vi "HipEXO_SM_R.vi"(10 "Trigger Ratio":dbl, 11 "Hip Angle":dbl) -> (1 "Flexion":bool, 2 "Extension":bool, 3 "ROM":dbl)   [LabVIEW 2018]
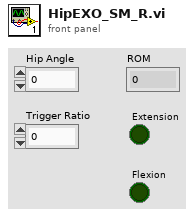
[diagram p1: front panel]
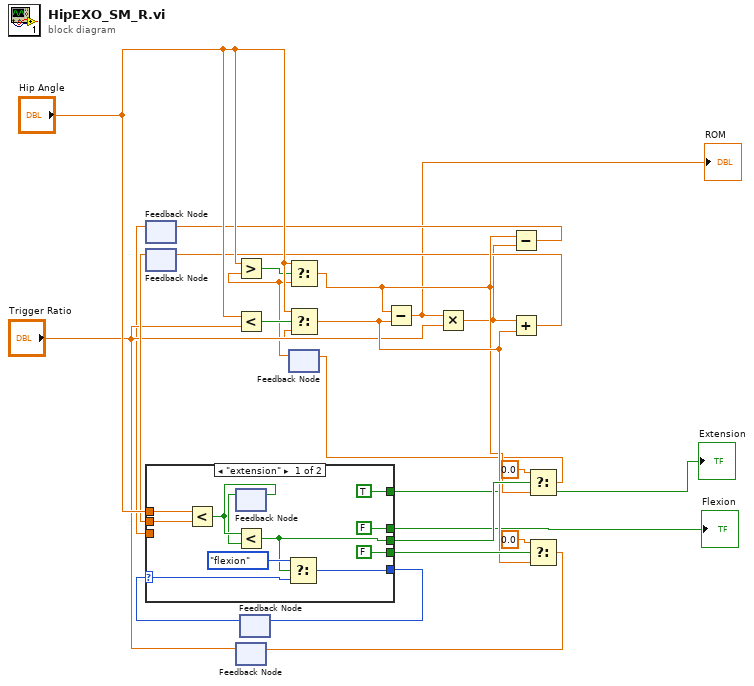
[diagram p0: block diagram]
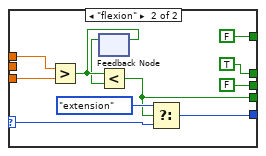
[diagram p2: hidden frame]
diagram:
  n1 = feedback #1() -> (w1:dbl)  [unwired: 1 in]
  n2 = feedback #2() -> (w16:dbl)  [unwired: 1 in]
  n3 = feedback #3() -> (w10:dbl)  [unwired: 1 in]
  n4 = Less?(x="Hip Angle", y=w10) -> (x < y?=w7:bool)
  n5 = feedback #4() -> (w3:enum16{"flexion", "extension"})  [unwired: 1 in]
  n6 = case shown="\"extension\"" w3 {
    selector: w3 -> [w32 w43]
    tunnel: [TRUE FALSE] -> w18
    tunnel: [w33 w44] -> w2
    tunnel: [FALSE TRUE] -> w19
    tunnel: "Hip Angle" -> [w30 w41]
    tunnel: w16 -> [w29 _]
    tunnel: w1 -> [_ w40]
    tunnel: [w25 FALSE ("output")] -> w22
    tunnel: [FALSE ("output") w36] -> w23
    frame "extension" {
      n7 = Less?(x=w30, y=w29) -> (x < y?=w27:bool)
      n8 = feedback-in #5(w27) -> ()
      n9 = feedback #5() -> (w26:bool)  [unwired: 1 in]
      n10 = Less?(x=w27, y=w26) -> (x < y?=w25:bool)
      n11 = Select(t=enum16{"flexion", "extension"}."flexion", s=w25, f=w32) -> (s? t:f=w33:enum16{"flexion", "extension"})
    }
    frame "flexion" {
      n12 = Greater?(x=w41, y=w40) -> (0:w38:bool)
      n13 = feedback-in #6(w38) -> ()
      n14 = feedback #6() -> (w37:bool)  [unwired: 1 in]
      n15 = Less?(x=w38, y=w37) -> (x < y?=w36:bool)
      n16 = Select(t=enum16{"flexion", "extension"}."extension", s=w36, f=w43) -> (s? t:f=w44:enum16{"flexion", "extension"})
    }
  }
  "Flexion" <- w19
  "Extension" <- w18
  n17 = feedback-in #4(w2) -> ()
  n18 = Select(t="Hip Angle", s=w7, f=w10) -> (s? t:f=w21:dbl)
  n19 = feedback #7() -> (w6:dbl)  [unwired: 1 in]
  n20 = Greater?(x="Hip Angle", y=w6) -> (0:w5:bool)
  n21 = Select(t="Hip Angle", s=w5, f=w6) -> (s? t:f=w20:dbl)
  n22 = Subtract(x=w20, y=w21) -> (x-y=w14:dbl)
  "ROM" <- w14
  n23 = Multiply(x=w14, y="Trigger Ratio") -> (x*y=w13:dbl)
  n24 = Subtract(x=w20, y=w13) -> (x-y=w17:dbl)
  n25 = feedback-in #1(w17) -> ()
  n26 = Add(x=w13, y=w21) -> (x+y=w15:dbl)
  n27 = feedback-in #2(w15) -> ()
  n28 = Select(t=0.0, s=w22, f=w20) -> (s? t:f=w11:dbl)
  n29 = feedback-in #7(w11) -> ()
  n30 = Select(t=0.0, s=w23, f=w21) -> (s? t:f=w9:dbl)
  n31 = feedback-in #3(w9) -> ()
